vi "Begin.vi"(8 "error in":errorcluster) -> (0 "error out":errorcluster)   [LabVIEW 2016]
doc: "Called before other user functions, this VI is expected to open initial I/O refnums, load in file data, and do all program initialization. Notice that the <B>error out</B> terminal is simply used for data flow. Wiring it to other structures or subVIs ensures that this VI runs first."
uses:
  <vilib>/Rock Robotics/SystemInterfaces/DIO/FPGA_DIOPWMChannel.ctl
  <vilib>/Rock Robotics/SystemInterfaces/DIO/FPGA_DIOChannel.ctl
  <vilib>/Rock Robotics/WPI/Joystick/WPI_JoystickDeviceEnum.ctl
  <vilib>/Rock Robotics/WPI/Solenoid/WPI_SolenoidChannel.ctl
  <vilib>/Rock Robotics/WPI/RobotDrive/WPI_RobotDriveOpen2MotorWithSPARK.vi
  <vilib>/Rock Robotics/WPI/Counter/WPI_CounterDigitalInputToDigitalSource.vi
  <vilib>/Rock Robotics/WPI/MotorControl/WPI_MotorControlOpen SPARK.vi
  <vilib>/Rock Robotics/WPI/Solenoid/WPI_SolenoidOpenSingle.vi
  Robot Global Data.vi
  <vilib>/Rock Robotics/WPI/ThirdParty/CanMotor/TalonSRX/WPI_CANTalonSRX_APIControlMode.ctl
  <vilib>/Rock Robotics/WPI/Solenoid/WPI_SolenoidOpenDouble.vi
  <vilib>/Rock Robotics/WPI/RobotDrive/WPI_RobotDriveOpen2MotorWithJaguar.vi
  <vilib>/Rock Robotics/WPI/MotorControl/WPI_MotorControlOpen Jaguar.vi
  <vilib>/Rock Robotics/WPI/RobotDrive/WPI_RobotDriveOpen4MotorWithSPARK.vi
  <vilib>/Rock Robotics/WPI/Switch/WPI_SwitchOpenLimit.vi
panel:
  in  "error in 2":errorcluster
  out "error out 2":errorcluster
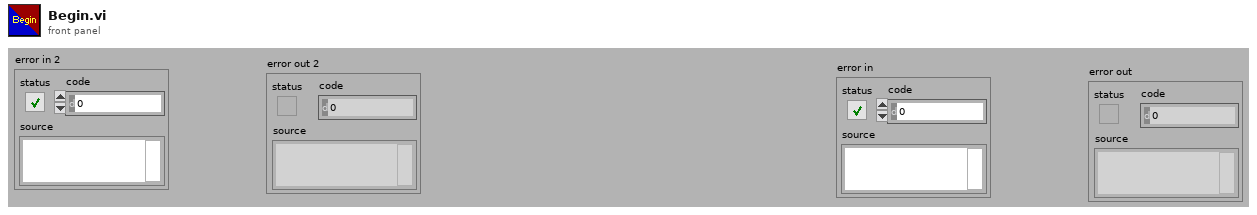
[diagram p1: front panel]
types:
  T1 = typedef "WPI_SolenoidChannel.ctl" = enum8{"Solenoid 0", "Solenoid 1", "Solenoid 2", "Solenoid 3", "Solenoid 4", "Solenoid 5", "Solenoid 6", "Solenoid 7", "Invalid"}
  T2 = typedef "FPGA_DIOChannel.ctl" = enum8{"DIO 0", "DIO 1", "DIO 2", "DIO 3", "DIO 4", "DIO 5", "DIO 6", "DIO 7", "DIO 8", "DIO 9", "DIO MXP 0", "DIO MXP 1", "DIO MXP 2", "DIO MXP 3", "DIO MXP 4", "DIO MXP 5", "DIO MXP 6", "DIO MXP 7", "DIO MXP 8", "DIO MXP 9", "DIO MXP 10", "DIO MXP 11", "DIO MXP 12", "DIO MXP 13", "DIO MXP 14", "DIO MXP 15", "SPI Port CS1", "SPI Port CS2", "SPI Port CS3", "SPI Port MISO", "SPI Port MOSI", "Invalid"}
  T3 = typedef "WPI_JoystickDeviceEnum.ctl" = enum16{"USB 0", "USB 1", "USB 2", "USB 3", "USB 4", "USB 5"}
  T4 = typedef "FPGA_DIOPWMChannel.ctl" = enum8{"PWM 0", "PWM 1", "PWM 2", "PWM 3", "PWM 4", "PWM 5", "PWM 6", "PWM 7", "PWM 8", "PWM 9", "PWM MXP 0", "PWM MXP 1", "PWM MXP 2", "PWM MXP 3", "PWM MXP 4", "PWM MXP 5", "PWM MXP 6", "PWM MXP 7", "PWM MXP 8", "PWM MXP 9", "Invalid"}
  T5 = typedef "WPI_JoystickDevRef.ctl" = cluster{"Device":T3}
  T6 = typedef "WPI_RobotDriveDevRef.ctl" = cluster{"DevStatus":errorcluster, "Motors[]":T7[], "Square Inputs":bool, "Max Output":dbl}
  T7 = typedef "WPI_MotorControlDeviceRef.ctl" = cluster{"DeviceStatus":errorcluster, "Type":T8, "PWM":cluster{"PWM Channel":T4, "DeadBand":T9}, "CAN":cluster{"Device Number":u8, "SetOutput VI Ref":variant, "GetOutput VI Ref":variant, "Enable VI Ref":variant, "Disable VI Ref":variant, "Data":variant}, "Invert":bool}
  T8 = typedef "WPI_MotorControlType.ctl" = enum16{"PWM", "CAN"}
  T9 = typedef "WPI_PWMDeadband.ctl" = cluster{"Name":string, "maxPositivePwm":i32, "minPositivePwm":i32, "centerPwm":i32, "maxNegativePwm":i32, "minNegativePwm":i32, "angularRange":u16}
  T10 = typedef "WPI_DigitalInputDevRef.ctl" = cluster{"DevStatus":errorcluster, "DIO Channel":T2}
  T11 = typedef "FPGA_CounterEncoderSourceConvertionLVSourceType.ctl" = cluster{"DevStatus":errorcluster, "AnalogTriggerMode?":bool, "DigitalMode":cluster{"DIO Channel":T12}, "AnalogTriggerMode":cluster{"AnalogTriggerIndex":T13, "OutputType":T14}}
  T12 = typedef "FPGA_DIODigitalSourceChannel.ctl" = enum8{"DIO 0", "DIO 1", "DIO 2", "DIO 3", "DIO 4", "DIO 5", "DIO 6", "DIO 7", "DIO 8", "DIO 9", "DIO MXP 0", "DIO MXP 1", "DIO MXP 2", "DIO MXP 3", "DIO MXP 4", "DIO MXP 5", "DIO MXP 6", "DIO MXP 7", "DIO MXP 8", "DIO MXP 9", "DIO MXP 10", "DIO MXP 11", "DIO MXP 12", "DIO MXP 13", "DIO MXP 14", "DIO MXP 15", "Disabled"}
  T13 = typedef "FPGA_AnalogTriggerIndex.ctl" = enum8{"Trig 0", "Trig 1", "Trig 2", "Trig 3", "Trig 4", "Trig 5", "Trig 6", "Trig 7", "Invalid"}
  T14 = typedef "FPGA_AnalogTriggerOutType.ctl" = enum16{"InWindow", "TriggerState", "Rising", "Falling"}
  T15 = typedef "WPI_EncoderDevRef.ctl" = cluster{"DevStatus":errorcluster, "EncoderIndex":T16, "CounterIndex":T17, "DistancePerCount":dbl, "Decoding Type":T18}
  T16 = typedef "FPGA_EncoderIdx.ctl" = enum8{"Enc 0", "Enc 1", "Enc 2", "Enc 3", "Enc 4", "Enc 5", "Enc 6", "Enc 7", "Invalid"}
  T17 = typedef "FPGA_CounterCtrSystemIndex.ctl" = enum8{"Ctr 0", "Ctr 1", "Ctr 2", "Ctr 3", "Ctr 4", "Ctr 5", "Ctr 6", "Ctr 7", "Invalid"}
  T18 = typedef "WPI_EncoderType.ctl" = enum16{"1x", "2x", "4x"}
  T19 = typedef "WPI_SolenoidDevRef.ctl" = cluster{"DevStatus":errorcluster, "Pneumatics Control Module":u8, "Forward Solenoid Channel":T1, "Reverse Solenoid Channel":T1}
  T20 = typedef "WPI_CANTalonSRX_APIControlMode.ctl" = enum8{"Percent VBus", "Speed", "Position", "Slave", "Unchanged / Invalid", "Voltage Compensation", "Current", "Motion Profile", "Motion Magic"}
  T21 = typedef "WPI_CameraDevRef.ctl" = cluster{"Camera Address":string, "CameraStatus":errorcluster}
  T22 = typedef "WPI_CompressorDevRef.ctl" = cluster{"DevStatus":errorcluster, "Pneumatics Control Module":u8}
  T23 = typedef "WPI_SwitchDevRef.ctl" = cluster{"DevStatus":errorcluster, "DIO Channel":T2, "CntIndex":T17, "Normally Closed":bool}
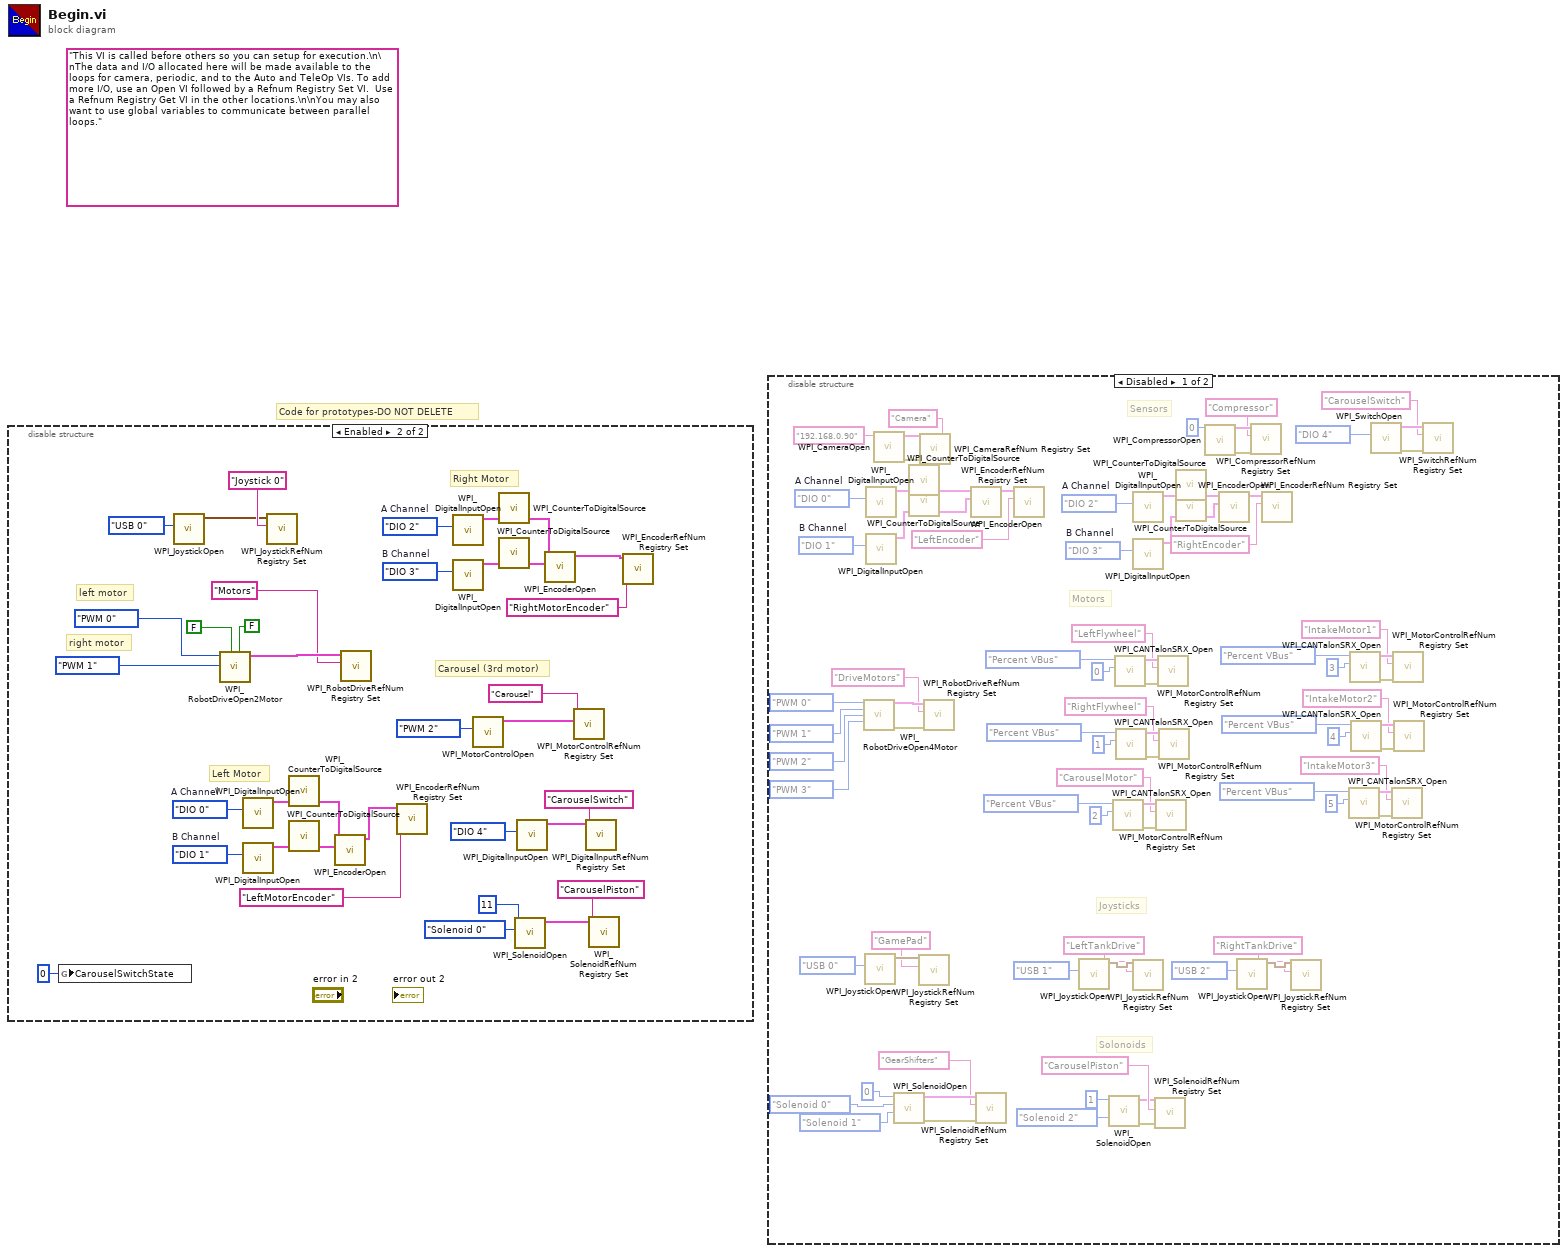
[diagram p0: block diagram]
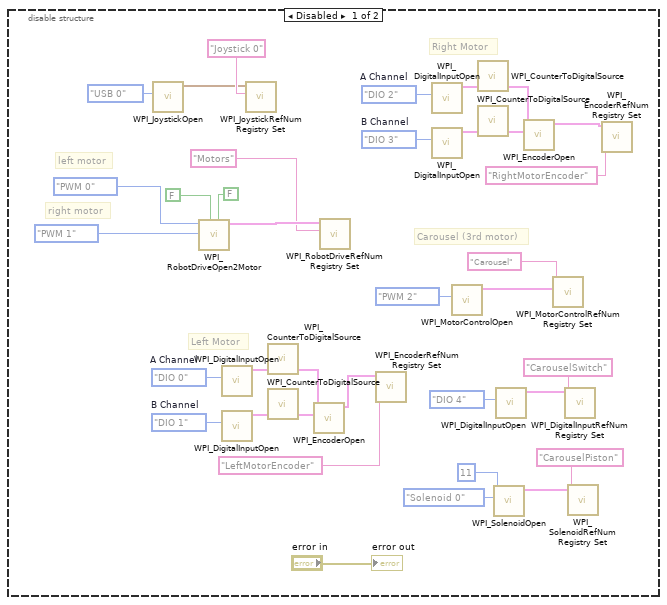
[diagram p3: hidden frame]
diagram:
  (unwired) "This VI is called before others so you can setup for execution.\n\nThe data and I/O allocated here will be made available to the loops for camera, periodic, and to the Auto and TeleOp VIs. To add more I/O, use an Open VI followed by a Refnum Registry Set VI.  Use a Refnum Registry Get VI in the other locations.\n\nYou may also want to use global variables to communicate between parallel loops."
  # "Code for prototypes-DO NOT DELETE"
  n1 = disable-structure shown="Enabled" {
    frame Disabled {
      w22 = FPGA_DIOChannel."DIO 3"  # B Channel
      w21 = FPGA_DIOChannel."DIO 2"  # A Channel
      w30 = FPGA_DIOChannel."DIO 1"  # B Channel
      w29 = FPGA_DIOChannel."DIO 0"  # A Channel
      # "Carousel (3rd motor)"
      # "Right Motor"
      # "right motor"
      # "left motor"
      # "Left Motor"
      n2 = call <vilib>:"WPI_JoystickOpen.vi"("JoystickDevice"=WPI_JoystickDeviceEnum."USB 0") -> ("JoystickDevRef"=w8:T5)  [unwired: 10 in]
      n3 = call-poly <vilib>:"WPI_RobotDriveOpen2Motor.vi"("Right Motor Inverted"=FALSE, "Left Motor Inverted"=FALSE, "Right Motor"=FPGA_DIOPWMChannel."PWM 1", "Left Motor"=FPGA_DIOPWMChannel."PWM 0") -> ("RobotDriveDevRef"=w32:T6)  [unwired: 6 in, 1 out]
      n4 = call <vilib>:"WPI_DigitalInputOpen.vi"("DIO Channel"=w29) -> ("DigitalInputDevRef"=w26:T10)  [unwired: 1 in, 9 out]
      n5 = call <vilib>:"WPI_DigitalInputOpen.vi"("DIO Channel"=w30) -> ("DigitalInputDevRef"=w27:T10)  [unwired: 1 in, 9 out]
      n6 = call <vilib>:"WPI_JoystickRefNum Registry Set.vi"("refnum name"="Joystick 0", "JoystickDevRef"=w8) -> ()  [unwired: 8 in, 2 out]
      n7 = call-poly <vilib>:"WPI_CounterToDigitalSource.vi"("DigitalInputDevRef"=w26) -> ("Digital Source"=w25:T11)  [unwired: 6 out]
      n8 = call-poly <vilib>:"WPI_CounterToDigitalSource.vi"("DigitalInputDevRef"=w27) -> ("Digital Source"=w28:T11)  [unwired: 6 out]
      n9 = call <vilib>:"WPI_EncoderOpen.vi"("BSource"=w28, "ASource"=w25) -> ("EncoderDevRef"=w24:T15)  [unwired: 6 in, 3 out]
      n10 = call <vilib>:"WPI_RobotDriveRefNum Registry Set.vi"("refnum name"="Motors", "RobotDriveDevRef"=w32) -> ()  [unwired: 8 in, 2 out]
      n11 = call <vilib>:"WPI_EncoderRefNum Registry Set.vi"("refnum name"="LeftMotorEncoder", "EncoderDevRef"=w24) -> ()  [unwired: 8 in, 2 out]
      n12 = call <vilib>:"WPI_DigitalInputOpen.vi"("DIO Channel"=w21) -> ("DigitalInputDevRef"=w18:T10)  [unwired: 1 in, 9 out]
      n13 = call <vilib>:"WPI_DigitalInputOpen.vi"("DIO Channel"=w22) -> ("DigitalInputDevRef"=w19:T10)  [unwired: 1 in, 9 out]
      n14 = call-poly <vilib>:"WPI_MotorControlOpen.vi"("PWM Channel"=FPGA_DIOPWMChannel."PWM 2") -> ("MotorControlDeviceRef"=w12:T7)  [unwired: 9 in, 1 out]
      n15 = call-poly <vilib>:"WPI_CounterToDigitalSource.vi"("DigitalInputDevRef"=w18) -> ("Digital Source"=w17:T11)  [unwired: 6 out]
      n16 = call-poly <vilib>:"WPI_CounterToDigitalSource.vi"("DigitalInputDevRef"=w19) -> ("Digital Source"=w20:T11)  [unwired: 6 out]
      n17 = call-poly <vilib>:"WPI_SolenoidOpen.vi"("Solenoid Channel"=WPI_SolenoidChannel."Solenoid 0", "Pneumatics Control Module (0)"=u8 11) -> ("SolenoidDevRef"=w4:T19)  [unwired: 8 in, 1 out]
      n18 = call <vilib>:"WPI_DigitalInputOpen.vi"("DIO Channel"=FPGA_DIOChannel."DIO 4") -> ("DigitalInputDevRef"=w6:T10)  [unwired: 9 in, 1 out]
      n19 = call <vilib>:"WPI_EncoderOpen.vi"("BSource"=w20, "ASource"=w17) -> ("EncoderDevRef"=w16:T15)  [unwired: 6 in, 3 out]
      n20 = call <vilib>:"WPI_MotorControlRefNum Registry Set.vi"("refnum name"="Carousel", "MotorControlDevRef"=w12) -> ()  [unwired: 8 in, 2 out]
      n21 = call <vilib>:"WPI_DigitalInputRefNum Registry Set.vi"("refnum name"="CarouselSwitch", "DigitalInputDevRef"=w6) -> ()  [unwired: 8 in, 2 out]
      n22 = call <vilib>:"WPI_SolenoidRefNum Registry Set.vi"("refnum name"="CarouselPiston", "SolenoidDevRef"=w4) -> ()  [unwired: 8 in, 2 out]
      n23 = call <vilib>:"WPI_EncoderRefNum Registry Set.vi"("refnum name"="RightMotorEncoder", "EncoderDevRef"=w16) -> ()  [unwired: 8 in, 2 out]
      "error out" <- "error in"
    }
    frame Enabled {
      w58 = FPGA_DIOChannel."DIO 3"  # B Channel
      w57 = FPGA_DIOChannel."DIO 2"  # A Channel
      w66 = FPGA_DIOChannel."DIO 1"  # B Channel
      w65 = FPGA_DIOChannel."DIO 0"  # A Channel
      # "Carousel (3rd motor)"
      # "Right Motor"
      # "right motor"
      # "left motor"
      # "Left Motor"
      n24 = global write "Robot Global Data.vi" "CarouselSwitchState"(u8 0 ("CarouselSwitchState")) -> ()
      n25 = call <vilib>:"WPI_JoystickOpen.vi"("JoystickDevice"=WPI_JoystickDeviceEnum."USB 0") -> ("JoystickDevRef"=w45:T5)  [unwired: 10 in]
      n26 = call-poly <vilib>:"WPI_RobotDriveOpen2Motor.vi"("Right Motor Inverted"=FALSE, "Left Motor Inverted"=FALSE, "Right Motor"=FPGA_DIOPWMChannel."PWM 1", "Left Motor"=FPGA_DIOPWMChannel."PWM 0") -> ("RobotDriveDevRef"=w68:T6)  [unwired: 6 in, 1 out]
      n27 = call <vilib>:"WPI_DigitalInputOpen.vi"("DIO Channel"=w65) -> ("DigitalInputDevRef"=w62:T10)  [unwired: 1 in, 9 out]
      n28 = call <vilib>:"WPI_DigitalInputOpen.vi"("DIO Channel"=w66) -> ("DigitalInputDevRef"=w63:T10)  [unwired: 1 in, 9 out]
      n29 = call <vilib>:"WPI_JoystickRefNum Registry Set.vi"("refnum name"="Joystick 0", "JoystickDevRef"=w45) -> ()  [unwired: 8 in, 2 out]
      n30 = call-poly <vilib>:"WPI_CounterToDigitalSource.vi"("DigitalInputDevRef"=w62) -> ("Digital Source"=w61:T11)  [unwired: 6 out]
      n31 = call-poly <vilib>:"WPI_CounterToDigitalSource.vi"("DigitalInputDevRef"=w63) -> ("Digital Source"=w64:T11)  [unwired: 6 out]
      n32 = call <vilib>:"WPI_EncoderOpen.vi"("BSource"=w64, "ASource"=w61) -> ("EncoderDevRef"=w60:T15)  [unwired: 6 in, 3 out]
      n33 = call <vilib>:"WPI_RobotDriveRefNum Registry Set.vi"("refnum name"="Motors", "RobotDriveDevRef"=w68) -> ()  [unwired: 8 in, 2 out]
      n34 = call <vilib>:"WPI_EncoderRefNum Registry Set.vi"("refnum name"="LeftMotorEncoder", "EncoderDevRef"=w60) -> ()  [unwired: 8 in, 2 out]
      n35 = call <vilib>:"WPI_DigitalInputOpen.vi"("DIO Channel"=w57) -> ("DigitalInputDevRef"=w54:T10)  [unwired: 1 in, 9 out]
      n36 = call <vilib>:"WPI_DigitalInputOpen.vi"("DIO Channel"=w58) -> ("DigitalInputDevRef"=w55:T10)  [unwired: 1 in, 9 out]
      n37 = call-poly <vilib>:"WPI_MotorControlOpen.vi"("PWM Channel"=FPGA_DIOPWMChannel."PWM 2") -> ("MotorControlDeviceRef"=w49:T7)  [unwired: 9 in, 1 out]
      n38 = call-poly <vilib>:"WPI_CounterToDigitalSource.vi"("DigitalInputDevRef"=w54) -> ("Digital Source"=w53:T11)  [unwired: 6 out]
      n39 = call-poly <vilib>:"WPI_CounterToDigitalSource.vi"("DigitalInputDevRef"=w55) -> ("Digital Source"=w56:T11)  [unwired: 6 out]
      n40 = call-poly <vilib>:"WPI_SolenoidOpen.vi"("Solenoid Channel"=WPI_SolenoidChannel."Solenoid 0", "Pneumatics Control Module (0)"=u8 11) -> ("SolenoidDevRef"=w41:T19)  [unwired: 8 in, 1 out]
      n41 = call <vilib>:"WPI_DigitalInputOpen.vi"("DIO Channel"=FPGA_DIOChannel."DIO 4") -> ("DigitalInputDevRef"=w43:T10)  [unwired: 9 in, 1 out]
      n42 = call <vilib>:"WPI_EncoderOpen.vi"("BSource"=w56, "ASource"=w53) -> ("EncoderDevRef"=w52:T15)  [unwired: 6 in, 3 out]
      n43 = call <vilib>:"WPI_MotorControlRefNum Registry Set.vi"("refnum name"="Carousel", "MotorControlDevRef"=w49) -> ()  [unwired: 8 in, 2 out]
      n44 = call <vilib>:"WPI_DigitalInputRefNum Registry Set.vi"("refnum name"="CarouselSwitch", "DigitalInputDevRef"=w43) -> ()  [unwired: 8 in, 2 out]
      n45 = call <vilib>:"WPI_SolenoidRefNum Registry Set.vi"("refnum name"="CarouselPiston", "SolenoidDevRef"=w41) -> ()  [unwired: 8 in, 2 out]
      n46 = call <vilib>:"WPI_EncoderRefNum Registry Set.vi"("refnum name"="RightMotorEncoder", "EncoderDevRef"=w52) -> ()  [unwired: 8 in, 2 out]
    }
  }
  n47 = disable-structure shown="Disabled" {
    frame Disabled {
      w136 = FPGA_DIOChannel."DIO 3"  # B Channel
      w135 = FPGA_DIOChannel."DIO 2"  # A Channel
      w144 = FPGA_DIOChannel."DIO 1"  # B Channel
      w143 = FPGA_DIOChannel."DIO 0"  # A Channel
      # "Solonoids"
      # "Joysticks"
      # "Motors"
      # "Sensors"
      n48 = call-poly <vilib>:"WPI_RobotDriveOpen4Motor.vi"("Rear Left Motor"=FPGA_DIOPWMChannel."PWM 0", "Rear Right Motor"=FPGA_DIOPWMChannel."PWM 1", "Front Left Motor"=FPGA_DIOPWMChannel."PWM 2", "Front Right Motor"=FPGA_DIOPWMChannel."PWM 3") -> ("RobotDriveDevRef"=w119:T6, "error out"=w120:errorcluster)  [unwired: 10 in]
      n49 = call <vilib>:"WPI_JoystickOpen.vi"("JoystickDevice"=WPI_JoystickDeviceEnum."USB 0") -> ("JoystickDevRef"=w157:T5)  [unwired: 10 in]
      n50 = call <vilib>:"WPI_DigitalInputOpen.vi"("DIO Channel"=w143) -> ("DigitalInputDevRef"=w140:T10)  [unwired: 1 in, 9 out]
      n51 = call <vilib>:"WPI_DigitalInputOpen.vi"("DIO Channel"=w144) -> ("DigitalInputDevRef"=w141:T10)  [unwired: 1 in, 9 out]
      n52 = call <vilib>:"WPI_CameraOpen.vi"("Camera Address"="192.168.0.90") -> ("error out"=w148:errorcluster, "CameraDevRef"=w147:T21)  [unwired: 9 in]
      n53 = call-poly <vilib>:"WPI_SolenoidOpen.vi"("Reverse Solenoid Channel"=WPI_SolenoidChannel."Solenoid 1", "Forward Solenoid Channel"=WPI_SolenoidChannel."Solenoid 0" ("Solenoid Channel"), "Pneumatics Control Module (0)"=u8 0) -> ("error out"=w128:errorcluster, "SolenoidDevRef"=w127:T19)  [unwired: 7 in]
      n54 = call-poly <vilib>:"WPI_CounterToDigitalSource.vi"("DigitalInputDevRef"=w140) -> ("Digital Source"=w139:T11)  [unwired: 6 out]
      n55 = call-poly <vilib>:"WPI_CounterToDigitalSource.vi"("DigitalInputDevRef"=w141) -> ("Digital Source"=w142:T11)  [unwired: 6 out]
      n56 = call <vilib>:"WPI_JoystickRefNum Registry Set.vi"("refnum name"="GamePad", "JoystickDevRef"=w157) -> ()  [unwired: 8 in, 2 out]
      n57 = call <vilib>:"WPI_CameraRefNum Registry Set.vi"("error in (no error)"=w148, "refnum name"="Camera", "CameraDevRef"=w147) -> ()  [unwired: 7 in, 2 out]
      n58 = call <vilib>:"WPI_RobotDriveRefNum Registry Set.vi"("error in (no error)"=w120, "refnum name"="DriveMotors", "RobotDriveDevRef"=w119) -> ()  [unwired: 7 in, 2 out]
      n59 = call <vilib>:"WPI_EncoderOpen.vi"("BSource"=w142, "ASource"=w139) -> ("EncoderDevRef"=w138:T15)  [unwired: 6 in, 3 out]
      n60 = call <vilib>:"WPI_SolenoidRefNum Registry Set.vi"("error in (no error)"=w128, "refnum name"="GearShifters", "SolenoidDevRef"=w127) -> ()  [unwired: 7 in, 2 out]
      n61 = call <vilib>:"WPI_EncoderRefNum Registry Set.vi"("refnum name"="LeftEncoder", "EncoderDevRef"=w138) -> ()  [unwired: 8 in, 2 out]
      n62 = call <vilib>:"WPI_JoystickOpen.vi"("JoystickDevice"=WPI_JoystickDeviceEnum."USB 1") -> ("JoystickDevRef"=w154:T5)  [unwired: 10 in]
      n63 = call-poly <vilib>:"WPI_SolenoidOpen.vi"("Solenoid Channel"=WPI_SolenoidChannel."Solenoid 2", "Pneumatics Control Module (0)"=u8 1) -> ("error out"=w76:errorcluster, "SolenoidDevRef"=w75:T19)  [unwired: 8 in]
      n64 = call <vilib>:"WPI_CANTalonSRX_Open.vi"("Device Number"=u8 2, "Control Mode"=WPI_CANTalonSRX_APIControlMode."Percent VBus") -> ("error out"=w99:errorcluster, "CAN Talon SRX Ref"=w98:T7)  [unwired: 8 in]
      n65 = call <vilib>:"WPI_CANTalonSRX_Open.vi"("Device Number"=u8 0, "Control Mode"=WPI_CANTalonSRX_APIControlMode."Percent VBus") -> ("error out"=w109:errorcluster, "CAN Talon SRX Ref"=w108:T7)  [unwired: 8 in]
      n66 = call <vilib>:"WPI_CANTalonSRX_Open.vi"("Device Number"=u8 1, "Control Mode"=WPI_CANTalonSRX_APIControlMode."Percent VBus") -> ("error out"=w104:errorcluster, "CAN Talon SRX Ref"=w103:T7)  [unwired: 8 in]
      n67 = call <vilib>:"WPI_DigitalInputOpen.vi"("DIO Channel"=w135) -> ("DigitalInputDevRef"=w132:T10)  [unwired: 1 in, 9 out]
      n68 = call <vilib>:"WPI_DigitalInputOpen.vi"("DIO Channel"=w136) -> ("DigitalInputDevRef"=w133:T10)  [unwired: 1 in, 9 out]
      n69 = call <vilib>:"WPI_JoystickRefNum Registry Set.vi"("refnum name"="LeftTankDrive", "JoystickDevRef"=w154) -> ()  [unwired: 8 in, 2 out]
      n70 = call <vilib>:"WPI_SolenoidRefNum Registry Set.vi"("error in (no error)"=w76, "refnum name"="CarouselPiston", "SolenoidDevRef"=w75) -> ()  [unwired: 7 in, 2 out]
      n71 = call <vilib>:"WPI_MotorControlRefNum Registry Set.vi"("error in (no error)"=w99, "refnum name"="CarouselMotor", "MotorControlDevRef"=w98) -> ()  [unwired: 7 in, 2 out]
      n72 = call <vilib>:"WPI_MotorControlRefNum Registry Set.vi"("error in (no error)"=w109, "refnum name"="LeftFlywheel", "MotorControlDevRef"=w108) -> ()  [unwired: 7 in, 2 out]
      n73 = call <vilib>:"WPI_MotorControlRefNum Registry Set.vi"("error in (no error)"=w104, "refnum name"="RightFlywheel", "MotorControlDevRef"=w103) -> ()  [unwired: 7 in, 2 out]
      n74 = call-poly <vilib>:"WPI_CounterToDigitalSource.vi"("DigitalInputDevRef"=w132) -> ("Digital Source"=w131:T11)  [unwired: 6 out]
      n75 = call-poly <vilib>:"WPI_CounterToDigitalSource.vi"("DigitalInputDevRef"=w133) -> ("Digital Source"=w134:T11)  [unwired: 6 out]
      n76 = call <vilib>:"WPI_CompressorOpen.vi"("Pneumatics Control Module (0)"=u8 0) -> ("CompressorDevRef"=w121:T22, "error out"=w122:errorcluster)  [unwired: 13 in]
      n77 = call <vilib>:"WPI_EncoderOpen.vi"("BSource"=w134, "ASource"=w131) -> ("EncoderDevRef"=w130:T15)  [unwired: 6 in, 3 out]
      n78 = call <vilib>:"WPI_JoystickOpen.vi"("JoystickDevice"=WPI_JoystickDeviceEnum."USB 2") -> ("JoystickDevRef"=w151:T5)  [unwired: 10 in]
      n79 = call <vilib>:"WPI_CompressorRefNum Registry Set.vi"("error in (no error)"=w122, "refnum name"="Compressor", "CompressorDevRef"=w121) -> ()  [unwired: 7 in, 2 out]
      n80 = call <vilib>:"WPI_EncoderRefNum Registry Set.vi"("refnum name"="RightEncoder", "EncoderDevRef"=w130) -> ()  [unwired: 8 in, 2 out]
      n81 = call <vilib>:"WPI_JoystickRefNum Registry Set.vi"("refnum name"="RightTankDrive", "JoystickDevRef"=w151) -> ()  [unwired: 8 in, 2 out]
      n82 = call <vilib>:"WPI_CANTalonSRX_Open.vi"("Device Number"=u8 5, "Control Mode"=WPI_CANTalonSRX_APIControlMode."Percent VBus") -> ("error out"=w84:errorcluster, "CAN Talon SRX Ref"=w83:T7)  [unwired: 8 in]
      n83 = call <vilib>:"WPI_CANTalonSRX_Open.vi"("Device Number"=u8 3, "Control Mode"=WPI_CANTalonSRX_APIControlMode."Percent VBus") -> ("error out"=w94:errorcluster, "CAN Talon SRX Ref"=w93:T7)  [unwired: 8 in]
      n84 = call <vilib>:"WPI_CANTalonSRX_Open.vi"("Device Number"=u8 4, "Control Mode"=WPI_CANTalonSRX_APIControlMode."Percent VBus") -> ("error out"=w89:errorcluster, "CAN Talon SRX Ref"=w88:T7)  [unwired: 8 in]
      n85 = call-poly <vilib>:"WPI_SwitchOpen.vi"("DIO Channel"=FPGA_DIOChannel."DIO 4") -> ("error out"=w81:errorcluster, "SwitchDevRef"=w80:T23)  [unwired: 9 in]
      n86 = call <vilib>:"WPI_MotorControlRefNum Registry Set.vi"("error in (no error)"=w84, "refnum name"="IntakeMotor3", "MotorControlDevRef"=w83) -> ()  [unwired: 7 in, 2 out]
      n87 = call <vilib>:"WPI_MotorControlRefNum Registry Set.vi"("error in (no error)"=w94, "refnum name"="IntakeMotor1", "MotorControlDevRef"=w93) -> ()  [unwired: 7 in, 2 out]
      n88 = call <vilib>:"WPI_MotorControlRefNum Registry Set.vi"("error in (no error)"=w89, "refnum name"="IntakeMotor2", "MotorControlDevRef"=w88) -> ()  [unwired: 7 in, 2 out]
      n89 = call <vilib>:"WPI_SwitchRefNum Registry Set.vi"("error in (no error)"=w81, "refnum name"="CarouselSwitch", "SwitchDevRef"=w80) -> ()  [unwired: 7 in, 2 out]
    }
    frame Enabled {
    }
  }
